vi "Sweep(Sub).vi"(0 "File":path, 1 "Low Frequency":dbl=200.0, 2 "High Frequency":dbl=1000.0, 3 "Time (s)":i32=10, 4 "Sample":i32=10000) -> (6 "Data":dbl[](array[numeric]))   [LabVIEW 2020]
uses:
  <vilib>/Analysis/NI_AALBase.lvlib
panel:
  out "Waveform Graph":waveform(dbl)(graph)
  out "Array Size":i32
  out "Data 2":dbl[](array[numeric])
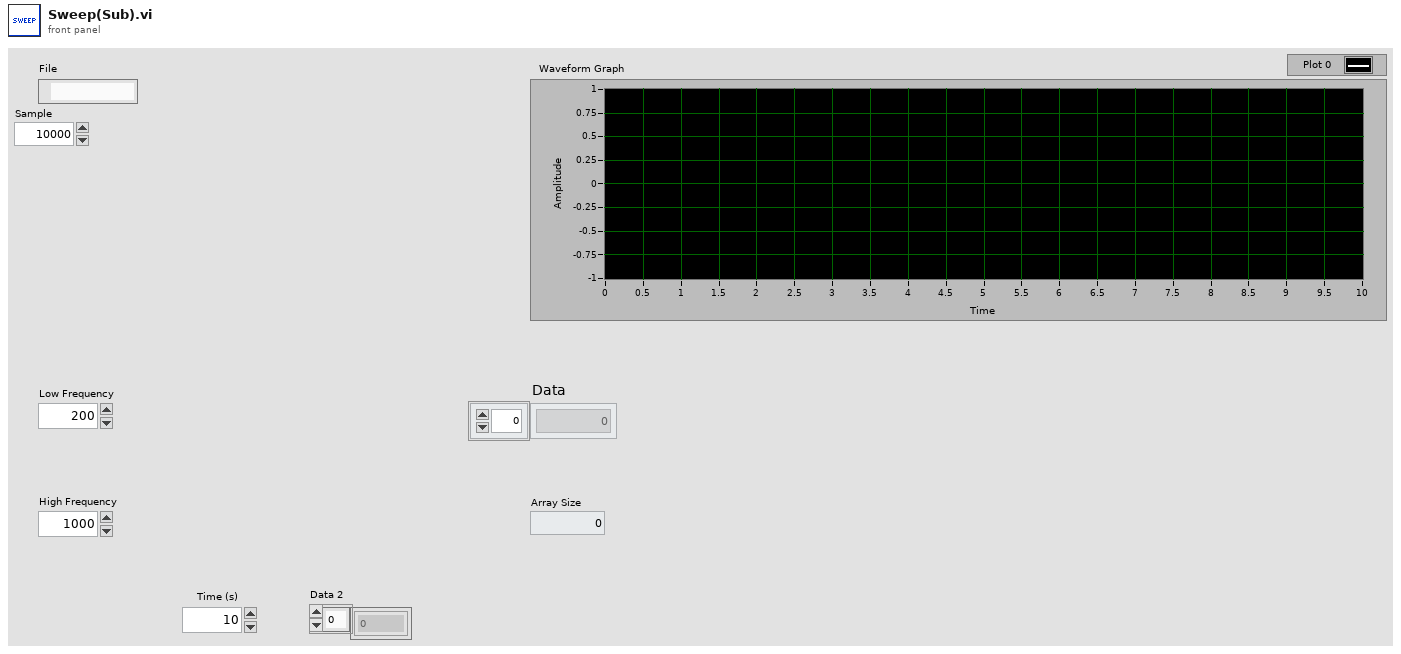
[diagram p1: front panel]
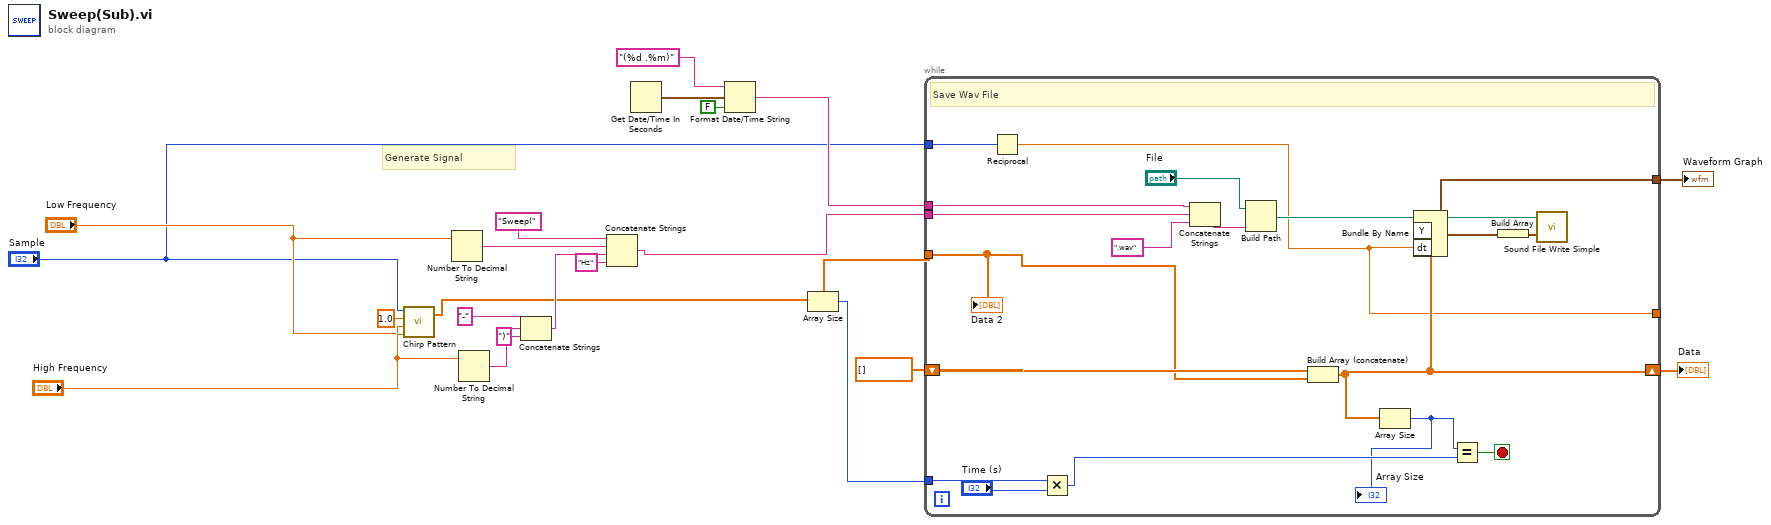
[diagram p0: block diagram]
diagram:
  # "Generate Signal"
  n1 = call <vilib>:"Chirp Pattern.vi"("f2"="High Frequency", "f1"="Low Frequency", "amplitude"=1.0, "samples"="Sample") -> ("Chirp Pattern"=w3:dbl[])  [unwired: 1 out]
  n2 = Number To Decimal String(number="Low Frequency") -> (decimal integer string=w16:string)  [unwired: 1 in]
  n3 = Number To Decimal String(number="High Frequency") -> (decimal integer string=w15:string)  [unwired: 1 in]
  n4 = Concatenate Strings("-" ("string"), w15, ")" ("string")) -> (w19:string)
  n5 = Concatenate Strings("Sweep(", w16, w19, "Hz" ("string")) -> (w9:string)
  n6 = Get Date/Time In Seconds() -> (seconds since 1Jan1904=w10:timestamp)
  n7 = Format Date/Time String(time format string (%c)="(%d .%m)", seconds (now)=w10, UTC format=FALSE) -> (date/time string=w13:string)
  n8 = Array Size(array=w3) -> (size(s)=w2:i32)
  n9 = while {
    tunnel: "Sample" -> [w39]
    tunnel: w3 -> [w36]
    shift-right: [w35] -> w8
    shift-left: dbl[] [] ("Array") -> [w37]
    tunnel: w2 -> [w31]
    tunnel: [w28] -> _
    tunnel: [w26] -> w7
    tunnel: w9 -> [w25]
    tunnel: w13 -> [w23]
    stop <- w34 stop-if-true
    # "Save Wav File"
    n10 = Reciprocal(x=w39) -> (1/x=w28:dbl)
    n11 = Multiply(x=w31, y="Time (s)") -> (x*y=w33:i32)
    n12 = Concatenate Strings(w23, w25, ".wav") -> (w27:string)
    n13 = Build Path(base path="File", name or relative path=w27) -> (appended path=w38:path)
    n14 = Build Array (concatenate)(w37, w36) -> (w35:dbl[])
    n15 = Array Size(array=w35) -> (size(s)=w32:i32)
    "Array Size" <- w32
    n16 = Bundle By Name("Y"=w35, "dt"=w28) -> (w26:waveform(dbl))  [unwired: 1 in]
    n17 = Equal?(x=w32, y=w33) -> (x = y?=w34:bool)
    n18 = Build Array(w26) -> (w29:waveform(dbl)[])
    n19 = call <vilib>:"Sound File Write Simple.vi"("data"=w29, "path"=w38) -> ()  [unwired: 8 in, 2 out]
    "Data 2" <- w36
  }
  "Data" <- w8
  "Waveform Graph" <- w7
